vi "IPS Read Current Sweep Rate.vi"(2 "Error In":errorcluster={"status"=FALSE, "code"=1073676294, "source"="VISA Read in Prologix USB GPIB Command.vi"}, 3 "VISA resource name (COM Port of Prologix Device)":refnum<visa-resource-name>="COM3") -> (0 "Error Out":errorcluster={"status"=FALSE, "code"=1073676294, "source"="VISA Read in Prologix_GPIB_Sample.vi"}, 1 "Sweep Rate (A/min)":dbl)   [LabVIEW 2011]
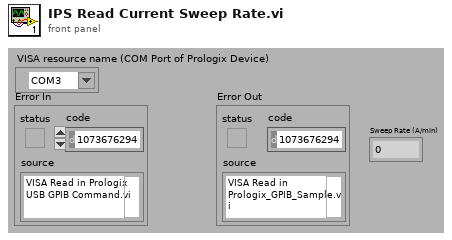
[diagram p1: front panel]
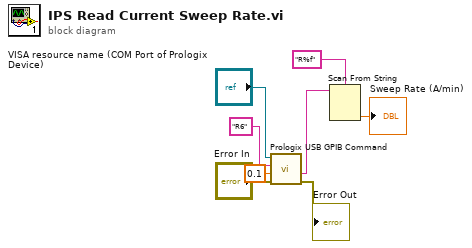
[diagram p0: block diagram]
diagram:
  n1 = call <userlib>:"Prologix USB GPIB Command.vi"("Error In"="Error In", "Wait for instrument to respond (s)"=0.1, "String to Send"="R6", "VISA resource name (COM Port of Prologix Device)"="VISA resource name (COM Port of Prologix Device)") -> ("Error Out"=→"Error Out":errorcluster, "Return String from Device (Not all commands return a String)"=w3:string)  [unwired: 2 out]
  n2 = Scan From String(format string="R%f", input string=w3) -> (output 1=→"Sweep Rate (A/min)":dbl)  [unwired: 2 in, 4 out]
